vi "SAOMM-HistoriqueEmulation.vi"(0 "Starting ID":u64=5685994523, 7 "Batch Size":i32=1) -> (4 "Last ID":u64=5685994524, 8 "FuckingHugeDataSet":u8[](array[numeric])=[28, 100, 233, 82, 1, 0, 0, 0, 86, 83, 130, 205, 0, 0, 0, 0, 0, 0, 0, 0, 0, 0, 0, 0, 0, 0, 0, 0, 0, 0, 0, 0, 0, 0, 0, 0, 0, 0, 0, 0, 1, 0, 0, 0, 0, 0, 0, 0, 0, 0, 0, 0, 0, 0, 0, 0, 0, 0, 0, 0, 0, 0, 0, 0, 0, 0, 0, 0, 0, 0, 0, 0, 0, 0, 0, 0, 0, 0, 0, 0, 0, 0, 0, 0, 0, 0, 0, 0, 0, 0, 0, 0, 0, 0, 0, 0, 0, 0, 0, 0, 0, 0, 0, 0, 0, 0, 0, 0, 0, 0, 0, 0, 0, 0, 0, 0, 0, 0, 0, 0, 0, 0, 0, 0, 0, 0, 0, 0, 0, 0, 0, 0, 0, 0, 0, 0, 0, 0, 0, 0, 0, 0, 0, 0, 0, 0, 0, 0, 0, 0, 0, 0, 0, 0, 0, 0, 0, 0, 0, 0, 0, 0, 0, 0, 0, 0, 0, 0, 0, 0, 0, 0, 0, 0, 0, 0, 0, 0, 0, 0, 0, 0, 0, 0, 0, 0, 0, 0, 0, 0, 0, 0, 0, 0, 0, 0, 0, 0, 0, 0, 0, 0, 0, 0, 0, 0, 0, 0, 0, 0, 0, 0, 0, 0, 0, 0, 0, 0, 0, 0, 0, 0, 0, 0, 0, 0, 0, 0, 0, 0, 0, 0, 0, 0, 0, 0, 0, 0, 0, 0, 0, 0, 0, 0, 0, 0, 0, 0, 0, 0, 0, 0, 0, 0, 0, 0, 0, 0, 0, 0, 0, 0, 0, 0, 0, 0, 0, 0, 0, 0, 0, 0, 0, 0, 0, 0, 0, 0, 0, 0, 0, 0, 0, 0, 0, 0, 0, 0, 0, 0, 0, 0, 0, 0, 0, 0, 0, 0, 0, 0, 0, 0, 0, 0, 0, 0, 0, 0, 0, 0, 0, 0, 0, 0, 0, 0, 0, 0, 0, 0, 0, 0, 0, 0, 0, 0, 0, 0, 0, 0, 0, 0, 0, 0, 0, 0, 0, 0, 0, 0, 0, 0, 0, 0, 0, 0, 0, 0, 0, 0, 0, 0, 0, 0, 0, 0, 0, 0, 0, 0, 0, 0, 0, 0, 0, 0, 0, 0, 0, 0, 0, 0])   [LabVIEW 2011]
uses:
  Polymorphics/Num2littleEndian(U64).vi
  Polymorphics/Num2littleEndian(DBL).vi
  Polymorphics/Num2littleEndian(U32).vi
panel:
  out "size(s)":i32=372
  out "length":i32=372
  in  "H_LUT V":dbl
  in  "H_LUT U":dbl
  in  "H_LUT Z":dbl
  in  "H_LUT Y":dbl
  in  "H_LUT X":dbl
  in  "Rotateur":dbl=3.0
  out "ID":u64=5685994524
  out "TimeStamp":u64=3447870294
  in  "Azimuth":dbl=1.0
  in  "Elevation":dbl=2.0
  in  "Mode":u32(ring)=1 items=["Opération Fixe", "Asservissement Ouvert", "Asservissement Fermé", "Calibration"]
  in  "H_Filtered V":dbl
  in  "H_Filtered U":dbl
  in  "H_Filtered Z":dbl
  in  "H_Filtered Y":dbl
  in  "H_Filtered X":dbl
  in  "Hv":dbl
  in  "Hu":dbl
  in  "Hz":dbl
  in  "Hy":dbl
  in  "Hx":dbl
  in  "H_Console V":dbl
  in  "H_Console U":dbl
  in  "H_Console Z":dbl
  in  "H_Console Y":dbl
  in  "H_Console X":dbl
  in  "H_Asser Y":dbl
  in  "H_Asser X":dbl
  in  "H_Offset V":dbl
  in  "H_Offset U":dbl
  in  "H_Offset Z":dbl
  in  "H_Offset Y":dbl
  in  "H_Offset X":dbl
  in  "H_Nominal V":dbl
  in  "H_Nominal U":dbl
  in  "H_Nominal Z":dbl
  in  "H_Nominal Y":dbl
  in  "H_Nominal X":dbl=16.0
  in  "Flux":dbl=11.0
  in  "Seuil du SNR":dbl=13.0
  in  "SNR":dbl=12.0
  in  "Centroïde Y":dbl=15.0
  in  "Centroïde X":dbl=14.0
  in  "Pixel de Référence Y":dbl=10.0
  in  "Pixel de Référence X":dbl=9.0
  in  "ROIWidth":u32=5
  in  "ROIHeight":u32=6
  in  "ROIXOffset":u32=7
  in  "ROIYOffset":u32=8
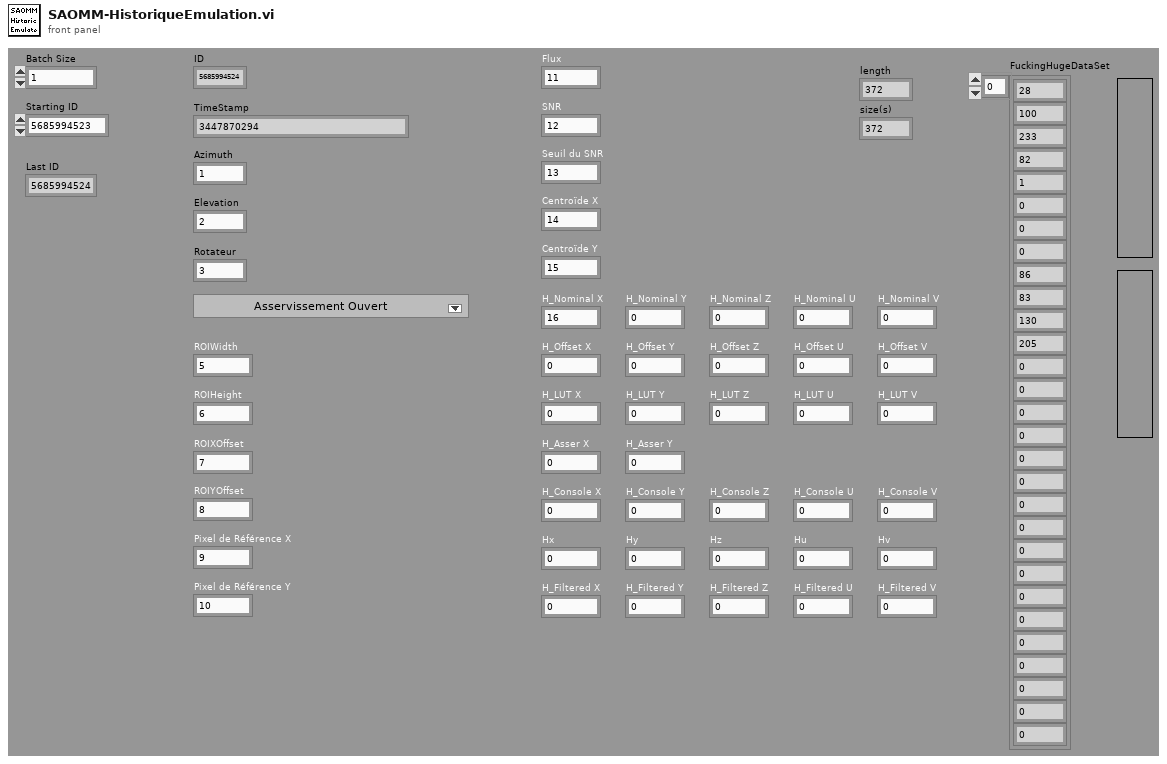
[diagram p1: front panel]
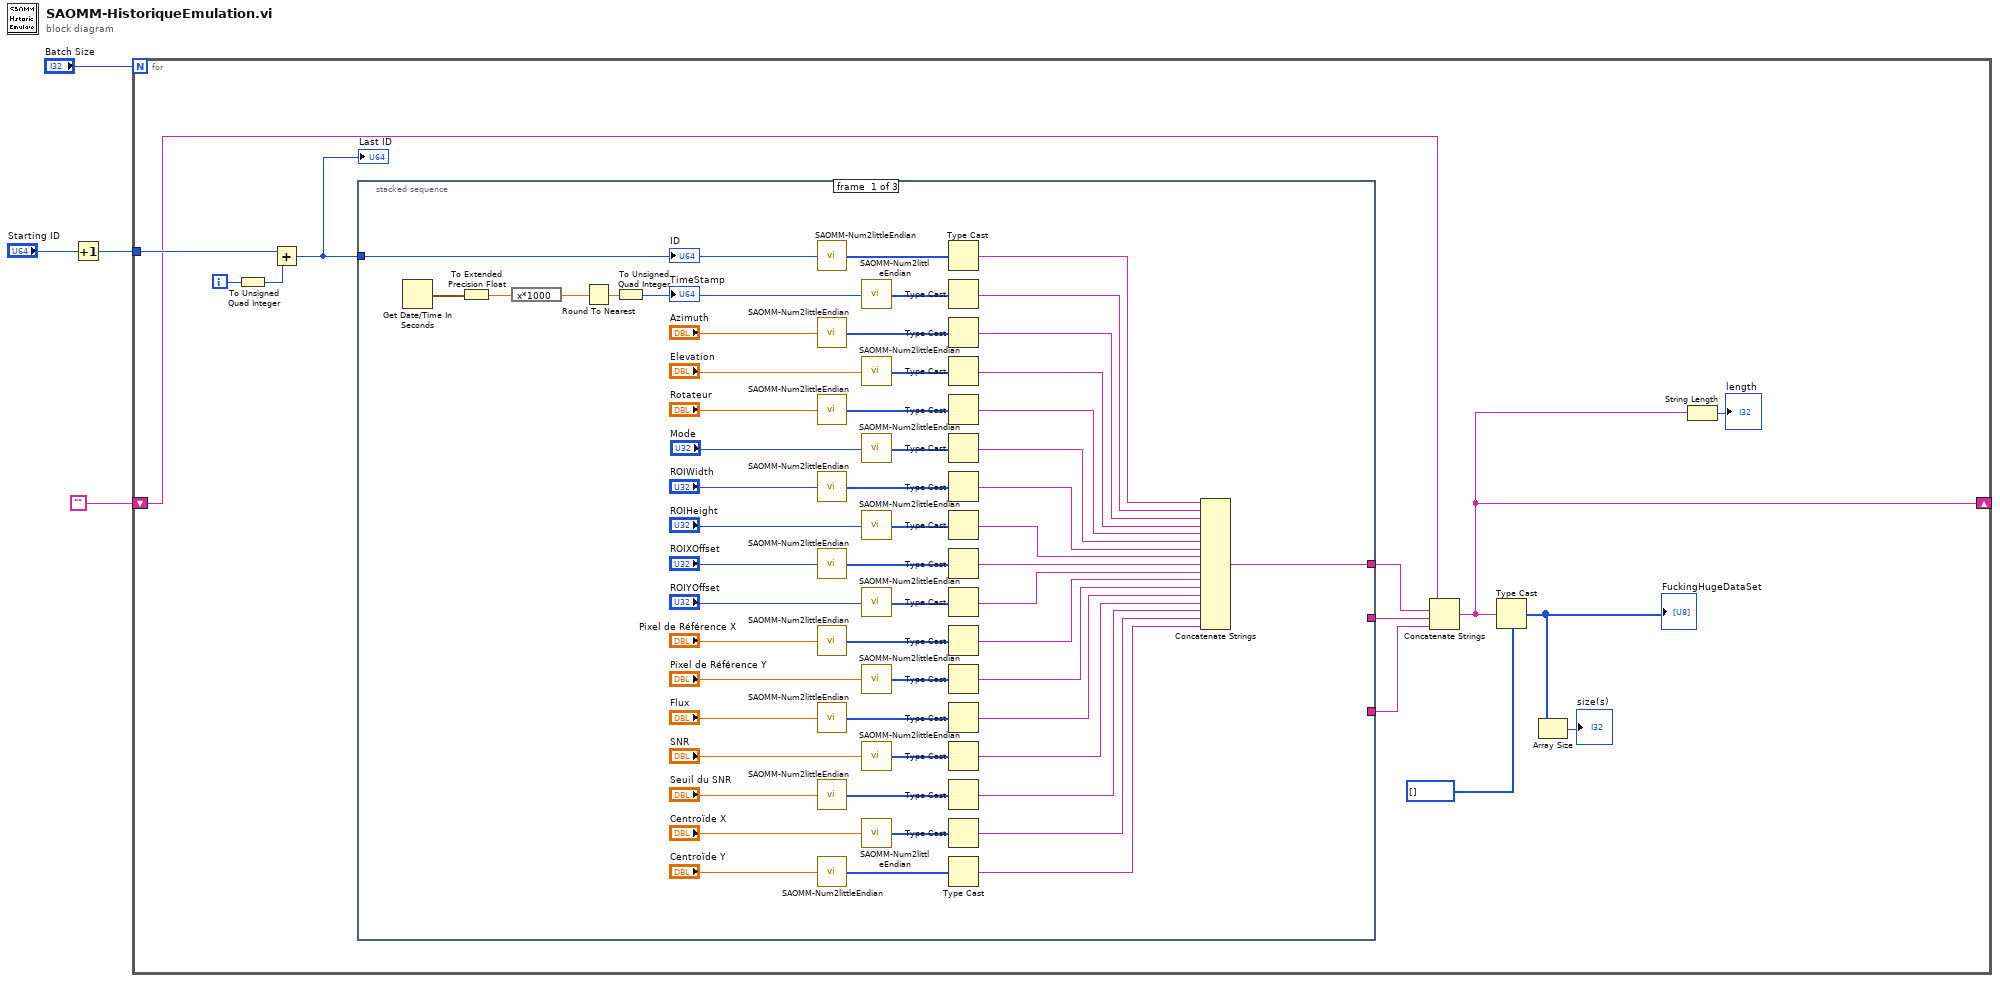
[diagram p0: block diagram]
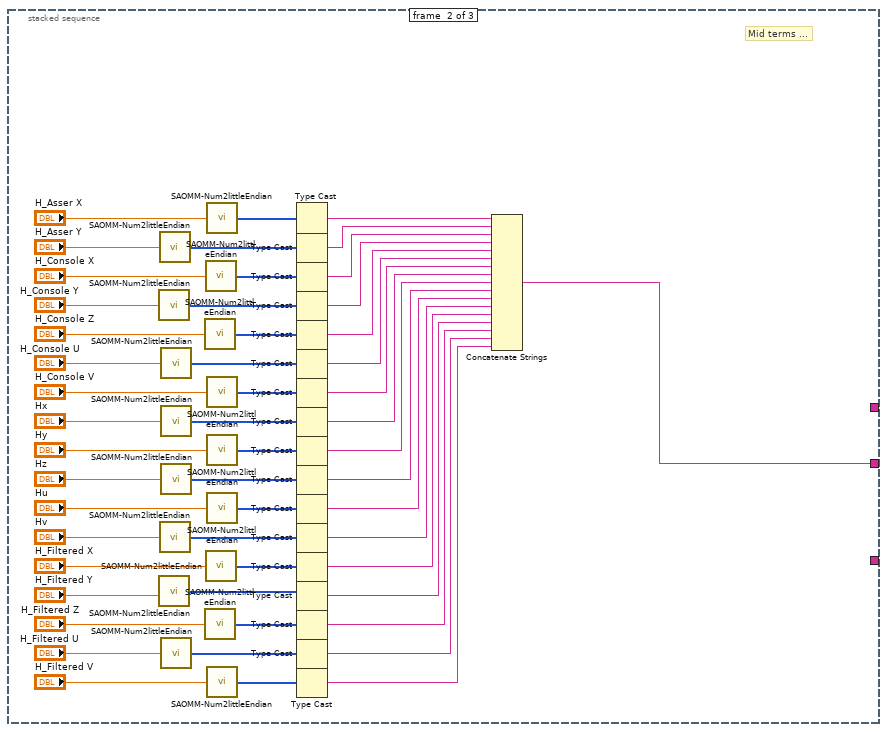
[diagram p2: hidden frame]
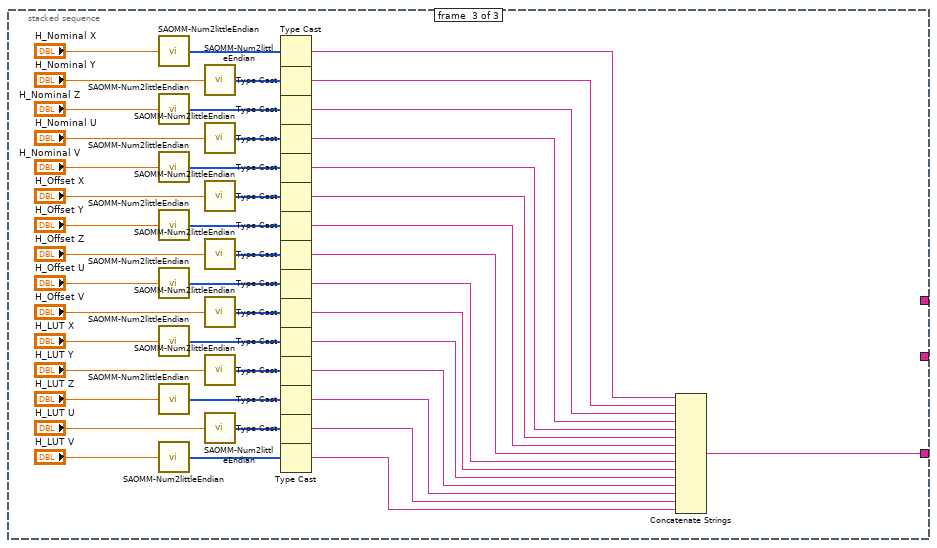
[diagram p3: hidden frame]
diagram:
  n1 = Increment(x="Starting ID") -> (x+1=w3:u64)
  n2 = for {
    N: "Batch Size" -> [_]
    tunnel: w3 -> [w17]
    shift-right: [w6] -> _
    shift-left: "" -> [w5]
    i -> [w16]
    n3 = To Unsigned Quad Integer(1:w16) -> (0:w15:u64)
    n4 = Add(x=w17, y=w15) -> (x+y=w7:u64)
    "Last ID" <- w7
    n5 = stacked-sequence {
      tunnel: w7 -> [w58 _ _]
      tunnel: [w23 _ _] -> w13
      tunnel: [_ w74 _] -> w14
      tunnel: [_ _ w126] -> w12
      frame #0 {
        n6 = Get Date/Time In Seconds() -> (seconds since 1Jan1904=w22:timestamp)
        n7 = To Extended Precision Float(1:w22) -> (0:w21:ext)
        n8 = expression code="x*1000"(w21) -> (w20:ext)
        n9 = Round To Nearest(number=w20) -> (nearest integer value=w19:ext)
        n10 = To Unsigned Quad Integer(1:w19) -> (0:w18:u64)
        "TimeStamp" <- w18
        n11 = call-poly "SAOMM-Num2littleEndian.vi"("Number"=w58) -> ("LiitleEndianedData"=w57:u8[])  [unwired: 14 in]
        n12 = call-poly "SAOMM-Num2littleEndian.vi"("Number"="Azimuth") -> ("LiitleEndianedData"=w55:u8[])  [unwired: 14 in]
        n13 = call-poly "SAOMM-Num2littleEndian.vi"("Number"="Rotateur") -> ("LiitleEndianedData"=w53:u8[])  [unwired: 14 in]
        n14 = call-poly "SAOMM-Num2littleEndian.vi"("Number"="ROIWidth") -> ("LiitleEndianedData"=w51:u8[])  [unwired: 14 in]
        n15 = call-poly "SAOMM-Num2littleEndian.vi"("Number"="ROIXOffset") -> ("LiitleEndianedData"=w49:u8[])  [unwired: 14 in]
        n16 = call-poly "SAOMM-Num2littleEndian.vi"("Number"="Pixel de Référence X") -> ("LiitleEndianedData"=w47:u8[])  [unwired: 14 in]
        n17 = call-poly "SAOMM-Num2littleEndian.vi"("Number"="Flux") -> ("LiitleEndianedData"=w45:u8[])  [unwired: 14 in]
        n18 = call-poly "SAOMM-Num2littleEndian.vi"("Number"="Seuil du SNR") -> ("LiitleEndianedData"=w43:u8[])  [unwired: 14 in]
        n19 = call-poly "SAOMM-Num2littleEndian.vi"("Number"="Centroïde Y") -> ("LiitleEndianedData"=w41:u8[])  [unwired: 14 in]
        n20 = call-poly "SAOMM-Num2littleEndian.vi"("Number"=w18) -> ("LiitleEndianedData"=w56:u8[])  [unwired: 14 in]
        n21 = call-poly "SAOMM-Num2littleEndian.vi"("Number"="Elevation") -> ("LiitleEndianedData"=w54:u8[])  [unwired: 14 in]
        n22 = call-poly "SAOMM-Num2littleEndian.vi"("Number"="Mode") -> ("LiitleEndianedData"=w52:u8[])  [unwired: 14 in]
        n23 = call-poly "SAOMM-Num2littleEndian.vi"("Number"="ROIHeight") -> ("LiitleEndianedData"=w50:u8[])  [unwired: 14 in]
        n24 = call-poly "SAOMM-Num2littleEndian.vi"("Number"="ROIYOffset") -> ("LiitleEndianedData"=w48:u8[])  [unwired: 14 in]
        n25 = call-poly "SAOMM-Num2littleEndian.vi"("Number"="Pixel de Référence Y") -> ("LiitleEndianedData"=w46:u8[])  [unwired: 14 in]
        n26 = call-poly "SAOMM-Num2littleEndian.vi"("Number"="SNR") -> ("LiitleEndianedData"=w44:u8[])  [unwired: 14 in]
        n27 = call-poly "SAOMM-Num2littleEndian.vi"("Number"="Centroïde X") -> ("LiitleEndianedData"=w42:u8[])  [unwired: 14 in]
        n28 = Type Cast(x=w57) -> (*(type *) &x=w40:string)  [unwired: 1 in]
        n29 = Type Cast(x=w56) -> (*(type *) &x=w39:string)  [unwired: 1 in]
        n30 = Type Cast(x=w55) -> (*(type *) &x=w38:string)  [unwired: 1 in]
        n31 = Type Cast(x=w54) -> (*(type *) &x=w37:string)  [unwired: 1 in]
        n32 = Type Cast(x=w53) -> (*(type *) &x=w36:string)  [unwired: 1 in]
        n33 = Type Cast(x=w52) -> (*(type *) &x=w35:string)  [unwired: 1 in]
        n34 = Type Cast(x=w51) -> (*(type *) &x=w34:string)  [unwired: 1 in]
        n35 = Type Cast(x=w50) -> (*(type *) &x=w33:string)  [unwired: 1 in]
        n36 = Type Cast(x=w49) -> (*(type *) &x=w32:string)  [unwired: 1 in]
        n37 = Type Cast(x=w48) -> (*(type *) &x=w31:string)  [unwired: 1 in]
        n38 = Type Cast(x=w47) -> (*(type *) &x=w30:string)  [unwired: 1 in]
        n39 = Type Cast(x=w46) -> (*(type *) &x=w29:string)  [unwired: 1 in]
        n40 = Type Cast(x=w45) -> (*(type *) &x=w28:string)  [unwired: 1 in]
        n41 = Type Cast(x=w44) -> (*(type *) &x=w27:string)  [unwired: 1 in]
        n42 = Type Cast(x=w43) -> (*(type *) &x=w26:string)  [unwired: 1 in]
        n43 = Type Cast(x=w42) -> (*(type *) &x=w25:string)  [unwired: 1 in]
        n44 = Type Cast(x=w41) -> (*(type *) &x=w24:string)  [unwired: 1 in]
        n45 = Concatenate Strings(w40, w39, w38, w37, w36, w35, w34, w33, w32, w31, w30, w29, w28, w27, w26, w25, w24) -> (w23:string)
        "ID" <- w58
      }
      frame #1 {
        # "Mid terms ..."
        n46 = call-poly "SAOMM-Num2littleEndian.vi"("Number"="H_Console Y") -> ("LiitleEndianedData"=w105:u8[])  [unwired: 14 in]
        n47 = call-poly "SAOMM-Num2littleEndian.vi"("Number"="H_Filtered Y") -> ("LiitleEndianedData"=w80:u8[])  [unwired: 14 in]
        n48 = call-poly "SAOMM-Num2littleEndian.vi"("Number"="H_Asser Y") -> ("LiitleEndianedData"=w107:u8[])  [unwired: 14 in]
        n49 = call-poly "SAOMM-Num2littleEndian.vi"("Number"="Hv") -> ("LiitleEndianedData"=w88:u8[])  [unwired: 14 in]
        n50 = call-poly "SAOMM-Num2littleEndian.vi"("Number"="H_Console U") -> ("LiitleEndianedData"=w103:u8[])  [unwired: 14 in]
        n51 = call-poly "SAOMM-Num2littleEndian.vi"("Number"="Hx") -> ("LiitleEndianedData"=w101:u8[])  [unwired: 14 in]
        n52 = call-poly "SAOMM-Num2littleEndian.vi"("Number"="Hz") -> ("LiitleEndianedData"=w99:u8[])  [unwired: 14 in]
        n53 = call-poly "SAOMM-Num2littleEndian.vi"("Number"="H_Filtered U") -> ("LiitleEndianedData"=w78:u8[])  [unwired: 14 in]
        n54 = call-poly "SAOMM-Num2littleEndian.vi"("Number"="H_Console Z") -> ("LiitleEndianedData"=w104:u8[])  [unwired: 14 in]
        n55 = call-poly "SAOMM-Num2littleEndian.vi"("Number"="H_Filtered Z") -> ("LiitleEndianedData"=w79:u8[])  [unwired: 14 in]
        n56 = call-poly "SAOMM-Num2littleEndian.vi"("Number"="H_Console X") -> ("LiitleEndianedData"=w106:u8[])  [unwired: 14 in]
        n57 = call-poly "SAOMM-Num2littleEndian.vi"("Number"="H_Filtered X") -> ("LiitleEndianedData"=w81:u8[])  [unwired: 14 in]
        n58 = call-poly "SAOMM-Num2littleEndian.vi"("Number"="H_Asser X") -> ("LiitleEndianedData"=w125:u8[])  [unwired: 14 in]
        n59 = call-poly "SAOMM-Num2littleEndian.vi"("Number"="H_Console V") -> ("LiitleEndianedData"=w102:u8[])  [unwired: 14 in]
        n60 = call-poly "SAOMM-Num2littleEndian.vi"("Number"="Hy") -> ("LiitleEndianedData"=w100:u8[])  [unwired: 14 in]
        n61 = call-poly "SAOMM-Num2littleEndian.vi"("Number"="Hu") -> ("LiitleEndianedData"=w98:u8[])  [unwired: 14 in]
        n62 = call-poly "SAOMM-Num2littleEndian.vi"("Number"="H_Filtered V") -> ("LiitleEndianedData"=w82:u8[])  [unwired: 14 in]
        n63 = Type Cast(x=w125) -> (*(type *) &x=w76:string)  [unwired: 1 in]
        n64 = Type Cast(x=w107) -> (*(type *) &x=w75:string)  [unwired: 1 in]
        n65 = Type Cast(x=w106) -> (*(type *) &x=w97:string)  [unwired: 1 in]
        n66 = Type Cast(x=w105) -> (*(type *) &x=w96:string)  [unwired: 1 in]
        n67 = Type Cast(x=w104) -> (*(type *) &x=w95:string)  [unwired: 1 in]
        n68 = Type Cast(x=w103) -> (*(type *) &x=w94:string)  [unwired: 1 in]
        n69 = Type Cast(x=w102) -> (*(type *) &x=w93:string)  [unwired: 1 in]
        n70 = Type Cast(x=w101) -> (*(type *) &x=w92:string)  [unwired: 1 in]
        n71 = Type Cast(x=w100) -> (*(type *) &x=w91:string)  [unwired: 1 in]
        n72 = Type Cast(x=w99) -> (*(type *) &x=w90:string)  [unwired: 1 in]
        n73 = Type Cast(x=w98) -> (*(type *) &x=w89:string)  [unwired: 1 in]
        n74 = Type Cast(x=w88) -> (*(type *) &x=w87:string)  [unwired: 1 in]
        n75 = Type Cast(x=w81) -> (*(type *) &x=w86:string)  [unwired: 1 in]
        n76 = Type Cast(x=w80) -> (*(type *) &x=w85:string)  [unwired: 1 in]
        n77 = Type Cast(x=w79) -> (*(type *) &x=w84:string)  [unwired: 1 in]
        n78 = Type Cast(x=w78) -> (*(type *) &x=w83:string)  [unwired: 1 in]
        n79 = Type Cast(x=w82) -> (*(type *) &x=w77:string)  [unwired: 1 in]
        n80 = Concatenate Strings(w76, w75, w97, w96, w95, w94, w93, w92, w91, w90, w89, w87, w86, w85, w84, w83, w77) -> (w74:string)
      }
      frame #2 {
        n81 = call-poly "SAOMM-Num2littleEndian.vi"("Number"="H_Nominal X") -> ("LiitleEndianedData"=w156:u8[])  [unwired: 14 in]
        n82 = call-poly "SAOMM-Num2littleEndian.vi"("Number"="H_Nominal Z") -> ("LiitleEndianedData"=w153:u8[])  [unwired: 14 in]
        n83 = call-poly "SAOMM-Num2littleEndian.vi"("Number"="H_Nominal V") -> ("LiitleEndianedData"=w151:u8[])  [unwired: 14 in]
        n84 = call-poly "SAOMM-Num2littleEndian.vi"("Number"="H_Offset Y") -> ("LiitleEndianedData"=w149:u8[])  [unwired: 14 in]
        n85 = call-poly "SAOMM-Num2littleEndian.vi"("Number"="H_Offset U") -> ("LiitleEndianedData"=w147:u8[])  [unwired: 14 in]
        n86 = call-poly "SAOMM-Num2littleEndian.vi"("Number"="H_LUT X") -> ("LiitleEndianedData"=w145:u8[])  [unwired: 14 in]
        n87 = call-poly "SAOMM-Num2littleEndian.vi"("Number"="H_LUT Z") -> ("LiitleEndianedData"=w143:u8[])  [unwired: 14 in]
        n88 = call-poly "SAOMM-Num2littleEndian.vi"("Number"="H_LUT V") -> ("LiitleEndianedData"=w141:u8[])  [unwired: 14 in]
        n89 = call-poly "SAOMM-Num2littleEndian.vi"("Number"="H_Nominal Y") -> ("LiitleEndianedData"=w154:u8[])  [unwired: 14 in]
        n90 = call-poly "SAOMM-Num2littleEndian.vi"("Number"="H_Nominal U") -> ("LiitleEndianedData"=w152:u8[])  [unwired: 14 in]
        n91 = call-poly "SAOMM-Num2littleEndian.vi"("Number"="H_Offset X") -> ("LiitleEndianedData"=w150:u8[])  [unwired: 14 in]
        n92 = call-poly "SAOMM-Num2littleEndian.vi"("Number"="H_Offset Z") -> ("LiitleEndianedData"=w148:u8[])  [unwired: 14 in]
        n93 = call-poly "SAOMM-Num2littleEndian.vi"("Number"="H_Offset V") -> ("LiitleEndianedData"=w146:u8[])  [unwired: 14 in]
        n94 = call-poly "SAOMM-Num2littleEndian.vi"("Number"="H_LUT Y") -> ("LiitleEndianedData"=w144:u8[])  [unwired: 14 in]
        n95 = call-poly "SAOMM-Num2littleEndian.vi"("Number"="H_LUT U") -> ("LiitleEndianedData"=w142:u8[])  [unwired: 14 in]
        n96 = Type Cast(x=w156) -> (*(type *) &x=w155:string)  [unwired: 1 in]
        n97 = Type Cast(x=w154) -> (*(type *) &x=w140:string)  [unwired: 1 in]
        n98 = Type Cast(x=w153) -> (*(type *) &x=w139:string)  [unwired: 1 in]
        n99 = Type Cast(x=w152) -> (*(type *) &x=w138:string)  [unwired: 1 in]
        n100 = Type Cast(x=w151) -> (*(type *) &x=w137:string)  [unwired: 1 in]
        n101 = Type Cast(x=w150) -> (*(type *) &x=w136:string)  [unwired: 1 in]
        n102 = Type Cast(x=w149) -> (*(type *) &x=w135:string)  [unwired: 1 in]
        n103 = Type Cast(x=w148) -> (*(type *) &x=w134:string)  [unwired: 1 in]
        n104 = Type Cast(x=w147) -> (*(type *) &x=w133:string)  [unwired: 1 in]
        n105 = Type Cast(x=w146) -> (*(type *) &x=w132:string)  [unwired: 1 in]
        n106 = Type Cast(x=w145) -> (*(type *) &x=w131:string)  [unwired: 1 in]
        n107 = Type Cast(x=w144) -> (*(type *) &x=w130:string)  [unwired: 1 in]
        n108 = Type Cast(x=w143) -> (*(type *) &x=w129:string)  [unwired: 1 in]
        n109 = Type Cast(x=w142) -> (*(type *) &x=w128:string)  [unwired: 1 in]
        n110 = Type Cast(x=w141) -> (*(type *) &x=w127:string)  [unwired: 1 in]
        n111 = Concatenate Strings(w155, w140, w139, w138, w137, w136, w135, w134, w133, w132, w131, w130, w129, w128, w127) -> (w126:string)
      }
    }
    n112 = Concatenate Strings(w5, w13, w14, w12) -> (w6:string)
    n113 = Type Cast(type=u8[] [], x=w6) -> (*(type *) &x=w10:u8[])
    "FuckingHugeDataSet" <- w10
    n114 = Array Size(array=w10) -> (size(s)=→"size(s)":i32)
    n115 = String Length(string=w6) -> (length=→"length":i32)
  }
